vi "Test Work Dispatcher Broadcast When Dispatching.vi"(8 "error in (no error)":errorcluster, 11 "Work Dispatcher Test in":refnum<class "Work Dispatcher Test.lvclass">=refnum) -> (0 "error out":errorcluster, 3 "Work Dispatcher Test out":refnum<class "Work Dispatcher Test.lvclass">)   [LabVIEW 2020, in "Work Dispatcher Test.lvclass"]
uses:
  Work Dispatcher Test.lvclass
  <vilib>/Astemes/Triarc Framework/Process/Process.lvclass
  Processes/Work Dispatcher/Work Dispatcher.lvclass
  C:/Program Files (x86)/National Instruments/LabVIEW 2020/vi.lib/Astemes/Triarc Framework/Process/Process.lvclass
  C:/Program Files (x86)/National Instruments/LabVIEW 2020/vi.lib/Astemes/Triarc Framework/Base/Base.lvclass
  C:/Program Files (x86)/National Instruments/LabVIEW 2020/vi.lib/Astemes/Triarc Framework/Error Handler Interface/Error Handler Interface.lvclass
  C:/Program Files (x86)/National Instruments/LabVIEW 2020/vi.lib/Astemes/Triarc Framework/Logging/Logging.lvclass
  C:/git/astemes-triarc-examples/source/Coffee Shop/Processes/Work Dispatcher/Work Dispatcher.lvclass
  C:/git/astemes-triarc-examples/source/Coffee Shop/Processes/People/Process Job/Job Handler.lvclass
  C:/Program Files (x86)/National Instruments/LabVIEW 2020/vi.lib/Astemes/Triarc Framework/Helper Loop/Helper Loop.lvclass
  <vilib>/Astemes/LUnit/Test Case.lvclass
  <vilib>/Astemes/Triarc Framework/Support/Broadcast Event Dequeuers.lvlib
  C:/Program Files (x86)/National Instruments/LabVIEW 2020/vi.lib/Astemes/LUnit/Test Case.lvclass
  C:/Program Files (x86)/National Instruments/LabVIEW 2020/vi.lib/Astemes/LUnit/LUnit Runnable.lvclass
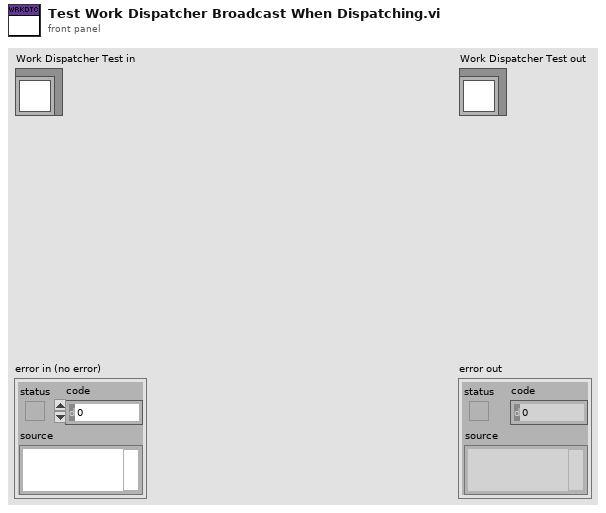
[diagram p1: front panel]
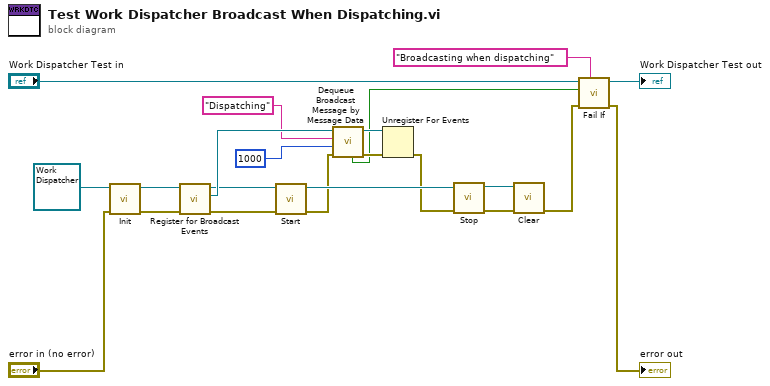
[diagram p0: block diagram]
diagram:
  n1 = call-dynamic "Init.vi"("error in (no error)"="error in (no error)", "Process In"=refnum<class "Work Dispatcher.lvclass"> refnum ("Work Dispatcher.lvclass")) -> ("error out"=w19:errorcluster, "Process Out"=w20:refnum<class "Work Dispatcher.lvclass">)  [unwired: 8 in]
  n2 = call <vilib>:"Register for Broadcast Events.vi"("error in (no error)"=w19, "Process In"=w20) -> ("error out"=w7:errorcluster, "Event Registration Refnum Out"=w15:refnum<event-registration>, "Process Out"=w8:refnum<class "Work Dispatcher.lvclass">)  [unwired: 7 in]
  n3 = call <vilib>:"Start.vi"("error in (no error)"=w7, "Process In"=w8) -> ("error out"=w12:errorcluster, "Process Out"=w18:refnum<class "Work Dispatcher.lvclass">)  [unwired: 7 in, 1 out]
  n4 = call <vilib>:"Dequeue Broadcast Message by Message Data.vi"("error in (no error)"=w12, "Timeout (-1)"=1000, "Message Data"="Dispatching", "Event Registration Refnum"=w15) -> ("error out"=w11:errorcluster, "Event Registration Refnum Out"=w9:refnum<event-registration>, "Timed Out?"=w1:bool)  [unwired: 3 in, 2 out]
  n5 = Unregister For Events(event registration refnum=w9, error in=w11) -> (error out=w10:errorcluster)
  n6 = call <vilib>:"Stop.vi"("error in (no error)"=w10, "Process In"=w18) -> ("error out"=w16:errorcluster, "Process Out"=w17:refnum<class "Work Dispatcher.lvclass">)  [unwired: 7 in, 1 out]
  n7 = call-dynamic "Clear.vi"("error in (no error)"=w16, "Process In"=w17) -> ("error out"=w2:errorcluster)  [unwired: 9 in]
  n8 = call <vilib>:"Fail If.vi"("Description"="Broadcasting when dispatching", "error in (no error)"=w2, "Fail?"=w1, "LUnit Test Case In"="Work Dispatcher Test in") -> ("error out"=→"error out":errorcluster, "LUnit Test Case Out"=→"Work Dispatcher Test out":refnum<class "Test Case.lvclass">)  [unwired: 6 in]
